vi "Increment PtByPt.vi"(2 "initialize":bool, 3 "activate":bool) -> (0 "overflow":bool, 1 "counter":u32)   [LabVIEW 2020, in "NI_PtbyPt.lvlib"]
doc: "Increments <B>counter</B> by one each time the VI is called when <B>activate</B> is set to TRUE."
uses:
  <vilib>/ptbypt/NI_PtbyPt.lvlib
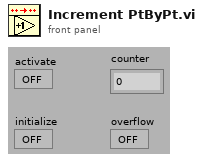
[diagram p1: front panel]
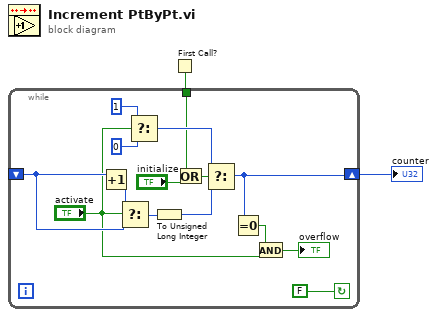
[diagram p0: block diagram]
diagram:
  n1 = First Call?() -> (First Call?: T/F=w1:bool)
  n2 = while {
    tunnel: w1 -> [w3]
    shift-left: _ -> [w15]
    shift-right: [w12] -> w2
    stop <- FALSE continue-if-true
    n3 = Increment(x=w15) -> (x+1=w17:u32)
    n4 = Select(t=w17, s="activate", f=w15) -> (s? t:f=w16:u32)
    n5 = Select(t=u32 1, s="activate", f=u32 0) -> (s? t:f=w7:u32)
    n6 = To Unsigned Long Integer(number=w16) -> (unsigned 32bit integer=w14:u32)
    n7 = Or(x=w3, y="initialize") -> (x .or. y?=w5:bool)
    n8 = Select(t=w7, s=w5, f=w14) -> (s? t:f=w12:u32)
    n9 = Equal To 0?(x=w12) -> (x = 0?=w11:bool)
    n10 = And(x=w11, y="activate") -> (x .and. y?=→"overflow":bool)
  }
  "counter" <- w2
